vi "Get PE Semaphore.vi"(8 "error in (no error)":errorcluster, 11 "CFG Base in":refnum<class "CFG Base.lvclass">) -> (0 "error out":errorcluster, 3 "CFG Base out":refnum<class "CFG Base.lvclass">)   [LabVIEW 2023, in "HAL GOOP4.lvlib" / "CFG Base.lvclass"]
uses:
  CFG Base.lvclass
  CFG Base.lvclass/CFG Base.ctl
panel:
  out "semaphore":T1
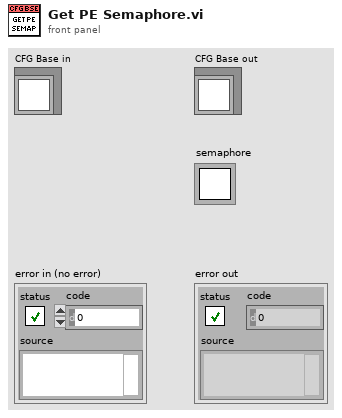
[diagram p1: front panel]
types:
  T1 = typedef "Semaphore RefNum" = refnum<k1>
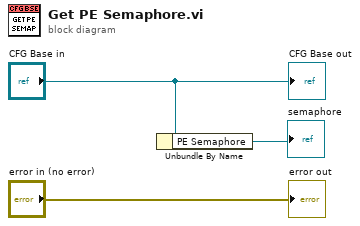
[diagram p0: block diagram]
diagram:
  n1 = Unbundle By Name("CFG Base in") -> ("PE Semaphore"=→"semaphore":T1)
  "error out" <- "error in (no error)"
  "CFG Base out" <- "CFG Base in"
